vi "期末-7.vi"() -> ()   [LabVIEW 2014]
uses:
  <vilib>/vision/NI_Vision_Development_Module.lvlib
panel:
  in  "紀錄電流":dbl[](array[numeric])
  in  "紀錄中點座標和":bool
  in  "Tab Control 2":enum32{"座標", "座標和", "作圖"}(tab)
  out "瞬間尖點座標":dbl[][](array[numeric])
  out "尖點座標和":dbl[](array[numeric])
  out "填入飽和磁場分量尖點座標和":dbl
  out "相減結果":dbl[](array[numeric])
  out "XY Graph":cluster{"紀錄電流":dbl[], dbl[]}(graph)
  in  "紀錄":bool
  in  "結束實驗":bool
  out "0. 原始畫面":T1(plugin-control)
  in  "1. 範圍選擇":T2={"色相（H）"={0, 255}, "飽和度（S）"={0, 255}, "亮度（L）"={0, 255}} {"亮度（L）" scale=0.0..255.0; "飽和度（S）" scale=0.0..255.0; "色相（H）" scale=0.0..255.0}
  out "Number of Particles":i32
  out "output cluster":cluster{"X":dbl, "Y":dbl}
  in  "Tab Control":T3(tab)
  out "1. 顏色選取":T1(plugin-control)
  out "2. 填補空隙":T1(plugin-control)
  out "4. 形狀修正":T1(plugin-control)
  out "5. 選取結果":T1(plugin-control)
  out "Particle Measurements":dbl[][](array[numeric])
  out "Error Out":errorcluster
  out "滑鼠位置顏色":T4
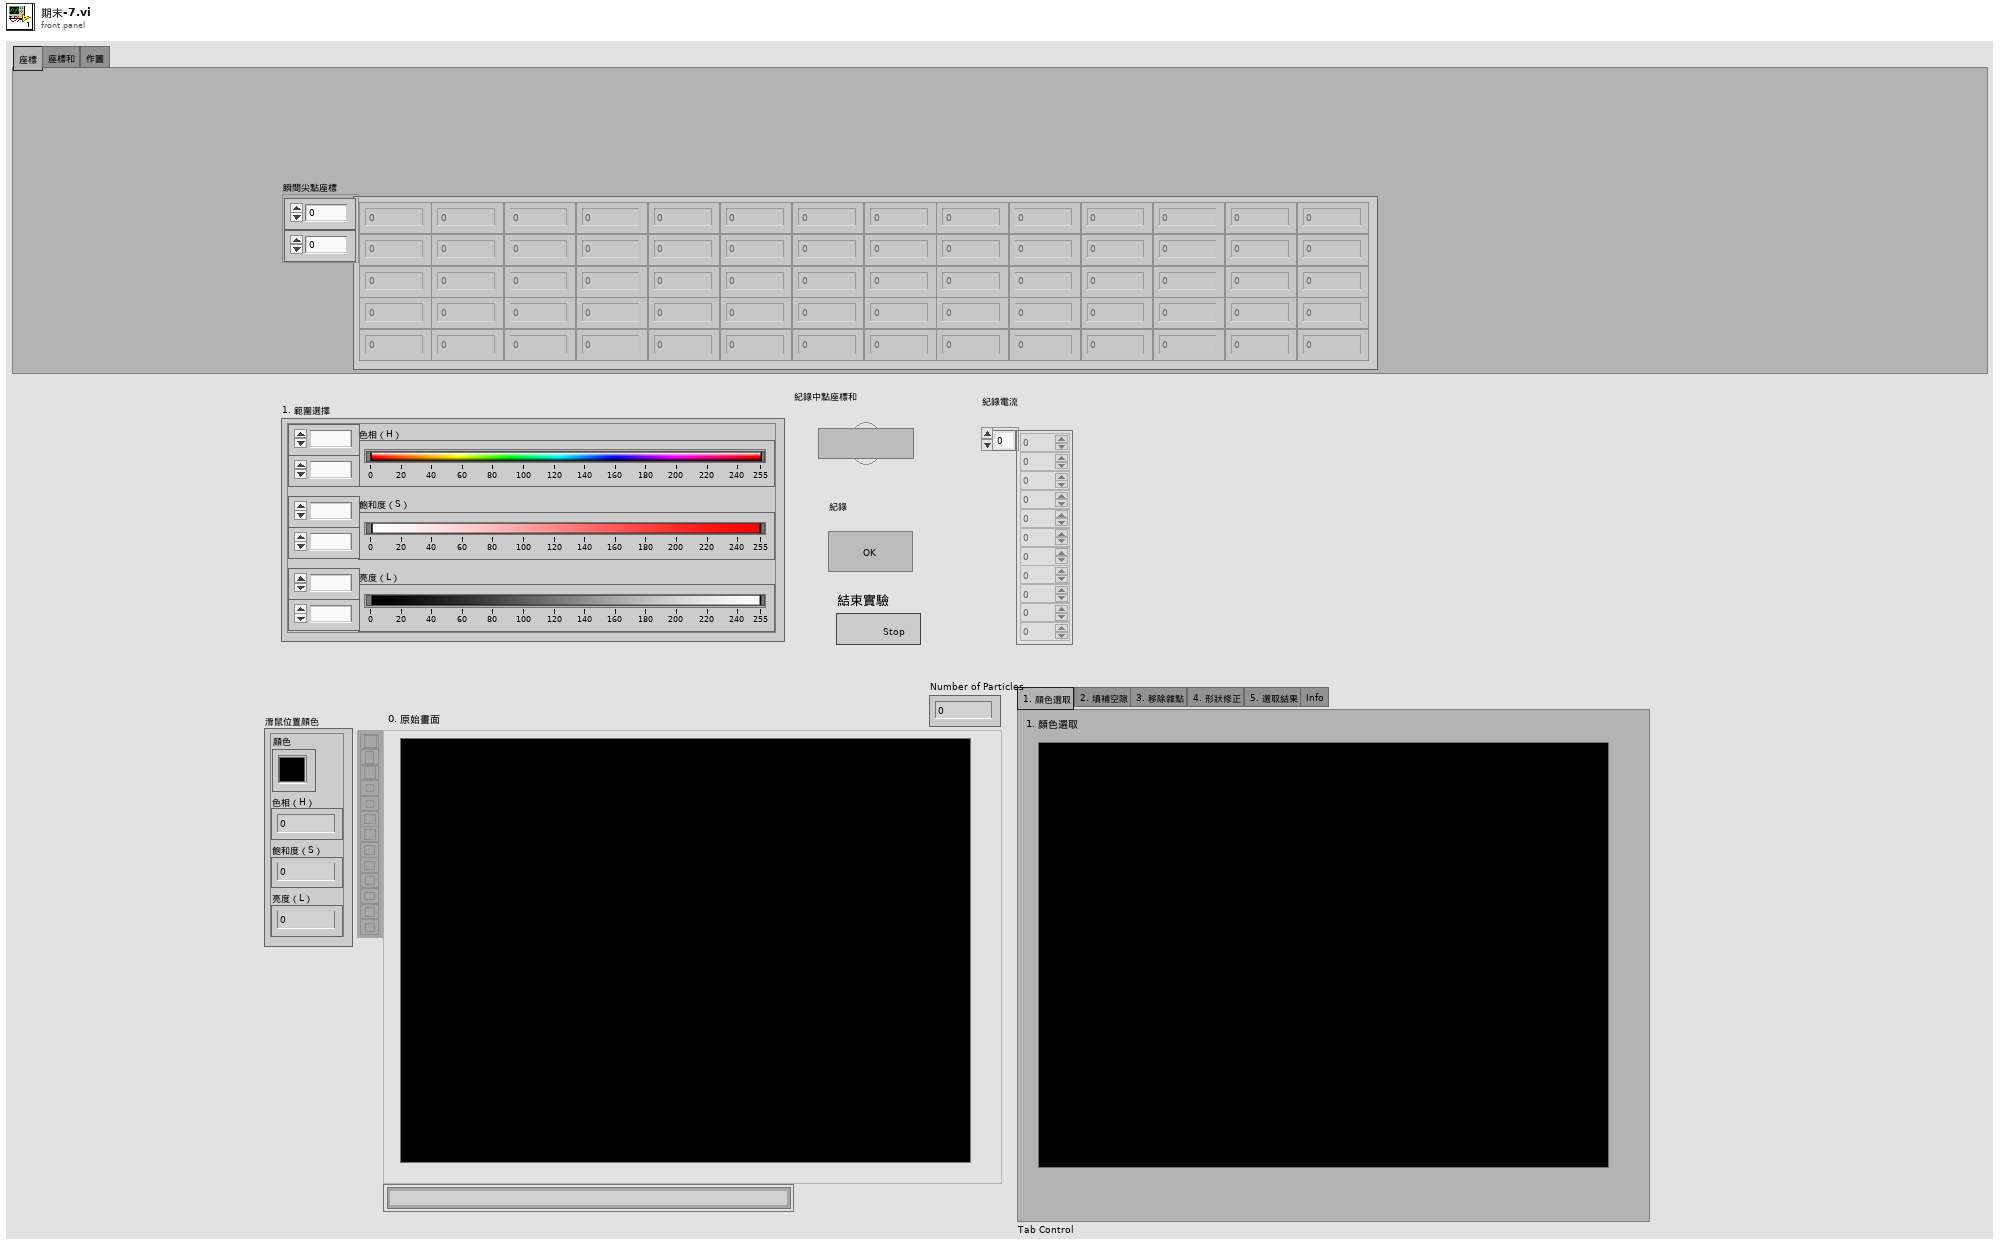
[diagram p1: front panel]
types:
  T1 = typedef "IMAQ Image.ctl" = refnum<image>
  T2 = cluster{"色相（H）":cluster{u8, u8}, "飽和度（S）":cluster{u8, u8}, "亮度（L）":cluster{u8, u8}}
  T3 = enum32{"1. 顏色選取", "2. 填補空隙", "3. 移除雜點", "4. 形狀修正", "5. 選取結果", "Info"}
  T4 = cluster{"色相（H）":u8, "飽和度（S）":u8, "亮度（L）":u8, "顏色":u32}
  T5 = cluster{"Numeric":dbl, "Numeric":dbl, "Numeric":dbl, "Numeric":dbl}
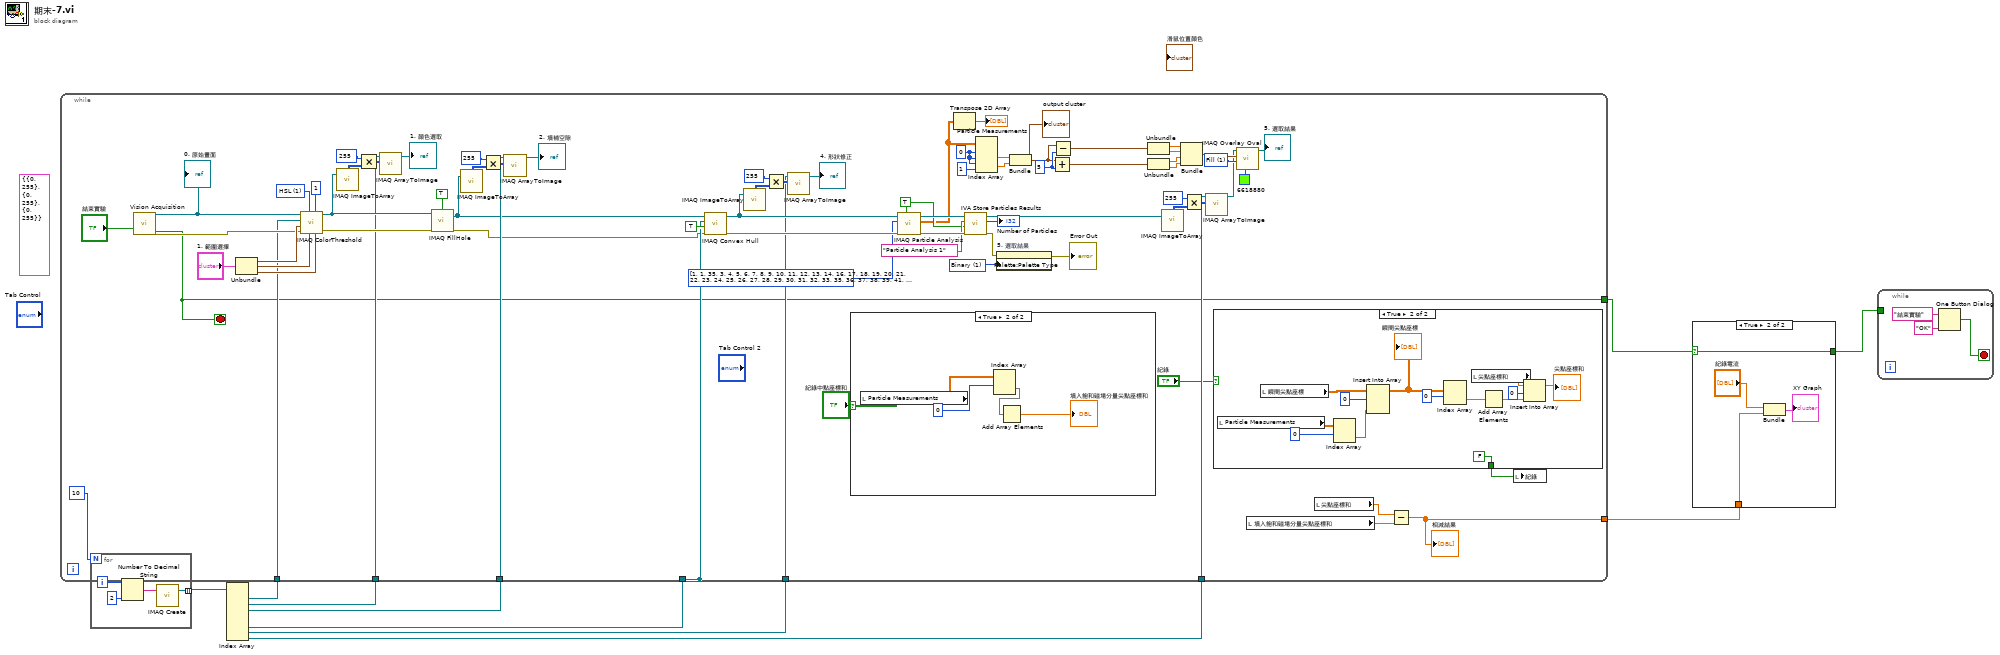
[diagram p0: block diagram]
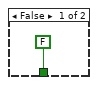
[diagram p4: hidden frame]
diagram:
  (unwired) T2 {"色相（H）"={0, 255}, "飽和度（S）"={0, 255}, "亮度（L）"={0, 255}} ("範圍選擇")
  n1 = for {
    N: 10 -> [_]
    tunnel: [w12] -> w11 mode=indexing
    i -> [w14]
    n2 = Number To Decimal String(number=w14, width (-)=2) -> (decimal integer string=w13:string)
    n3 = call "IMAQ Create"("Image Name"=w13) -> ("New Image"=w12:T1)  [unwired: 4 in, 1 out]
  }
  n4 = Index Array(array=w11) -> (element #1=w10:T1, element #2=w9:T1, element #3=w8:T1, element #6=w6:T1, element #7=w5:T1, element #8=w4:T1)  [unwired: 8 in, 2 out]
  n5 = while {
    tunnel: w8 -> [w58]
    tunnel: w6 -> [w69]
    tunnel: [w69] -> _
    tunnel: w9 -> [w63]
    tunnel: w10 -> [w57]
    tunnel: w5 -> [w51]
    tunnel: w4 -> [w28]
    tunnel: [w22] -> w3
    tunnel: [w16] -> w1
    stop <- w22 stop-if-true
    w33 = u32 1 items=["Frame", "Fill"] ("Drawing Mode (Frame)")
    w42 = 5
    w47 = 0
    w71 = u32 1 items=["Grayscale", "Binary", "Gradient", "Rainbow", "Temperature", "User Defined"] ("Palette")
    w76 = i32[] [1, 1, 35, 3, 4, 5, 6, 7, 8, 9, 10, 11, 12, 13, 14, 16, 17, 18, 19, 20, 21, 22, 23, 24, 25, 26, 27, 28, 29, 30, 31, 32, 33, 35, 36, 37, 38, 39, 41, 42, 43, 45, 46, 48, 49, 50, 51, 53, 54, 55, 56, 58, 59, 60, 61, 62, 63, 64, 65, 66, 68, 69, 70, 71, 72, 73, 74, 75, 76, 77, 78, 79, 80, 81, 82, 83, 84, 85, 86, 87, 88] items=["Center of Mass X", "Center of Mass Y", "First Pixel X", "First Pixel Y", "Bounding Rect Left", "Bounding Rect Top", "Bounding Rect Right", "Bounding Rect Bottom", "Max Feret Diameter Start X", "Max Feret Diameter Start Y", "Max Feret Diameter End X", "Max Feret Diameter End Y", "Max Horiz. Segment Length Left", "Max Horiz. Segment Length Right", "Max Horiz. Segment Length Row", "-", "Bounding Rect Width", "Bounding Rect Height", "Bounding Rect Diagonal", "Perimeter", "Convex Hull Perimeter", "Holes' Perimeter", "Max Feret Diameter", "Equivalent Ellipse Major Axis", "Equivalent Ellipse Minor Axis", "Equivalent Ellipse Minor Axis (Feret)", "Equivalent Rect Long Side", "Equivalent Rect Short Side", "Equivalent Rect Diagonal", "Equivalent Rect Short Side (Feret)", "Average Horiz. Segment Length", "Average Vert. Segment Length", "Hydraulic Radius", "Waddel Disk Diameter", "-", "Area", "Holes' Area", "Particle & Holes' Area", "Convex Hull Area", "Image Area", "-", "Number of Holes", "Number of Horiz. Segments", "Number of Vert. Segments", "-", "Orientation", "Max Feret Diameter Orientation", "-", "% Area/Image Area", "% Area/(Particle & Holes' Area)", "Ratio of Equivalent Ellipse Axes", "Ratio of Equivalent Rect Sides", "-", "Elongation Factor", "Compactness Factor", "Heywood Circularity Factor", "Type Factor", "-", "Sum X", "Sum Y", "Sum XX", "Sum XY", "Sum YY", "Sum XXX", "Sum XXY", "Sum XYY", "Sum YYY", "-", "Moment of Inertia XX", "Moment of Inertia XY", "Moment of Inertia YY", "Moment of Inertia XXX", "Moment of Inertia XXY", "Moment of Inertia XYY", "Moment of Inertia YYY", "Norm. Moment of Inertia XX", "Norm. Moment of Inertia XY", "Norm. Moment of Inertia YY", "Norm. Moment of Inertia XXX", "Norm. Moment of Inertia XXY", "Norm. Moment of Inertia XYY", "Norm. Moment of Inertia YYY", "Hu Moment 1", "Hu Moment 2", "Hu Moment 3", "Hu Moment 4", "Hu Moment 5", "Hu Moment 6", "Hu Moment 7"] ("Pixel Measurements")
    w78 = TRUE ("Connectivity 4/8 (8)")
    w87 = u16 1 items=["RGB", "HSL", "HSV", "HSI"] ("Color Mode")
    n6 = call "Vision Acquisition"("Stop (F)"="結束實驗") -> ("Image Out"=w89:T1, "Stopped"=w22:bool, "error out"=w82:errorcluster)  [unwired: 24 in]
    "0. 原始畫面" <- w89
    n7 = Unbundle("1. 範圍選擇") -> ("色相（H）"=w86:cluster{u8, u8}, "飽和度（S）"=w85:cluster{u8, u8}, "亮度（L）"=w84:cluster{u8, u8})
    n8 = call "IMAQ ColorThreshold"("Blue or Luma or Val or Inten Range"=w84, "Replace Value"=1, "Green or Sat Range"=w85, "Color Mode"=w87, "error in (no error)"=w82, "Red or Hue Range"=w86, "Image Dst"=w57, "Image Src"=w89) -> ("error out"=w73:errorcluster, "Image Dst Out"=w68:T1)  [unwired: 2 out]
    n9 = call "IMAQ ImageToArray"("Image"=w68) -> ("Image Pixels (U8)"=w66:u8[][])  [unwired: 3 in, 4 out]
    n10 = Multiply(x=255, y=w66) -> (x*y=w65:i32[][])
    n11 = call "IMAQ ArrayToImage"("Image Pixels (U8)"=w65, "Image"=w63) -> ("Image Out"=→"1. 顏色選取":T1)  [unwired: 8 in, 1 out]
    n12 = call "IMAQ FillHole"("error in (no error)"=w73, "Image Src"=w68, "Connectivity 4/8 (8)"=TRUE) -> ("error out"=w20:errorcluster, "Image Dst Out"=w21:T1)  [unwired: 1 in, 2 out]
    n13 = call "IMAQ ImageToArray"("Image"=w21) -> ("Image Pixels (U8)"=w61:u8[][])  [unwired: 3 in, 4 out]
    n14 = Multiply(x=255, y=w61) -> (x*y=w62:i32[][])
    n15 = call "IMAQ ArrayToImage"("Image Pixels (U8)"=w62, "Image"=w58) -> ("Image Out"=→"2. 填補空隙":T1)  [unwired: 8 in, 1 out]
    n16 = call "IMAQ Convex Hull"("error in (no error)"=w20, "Connectivity 4/8 (8)"=TRUE, "Image Dst"=w69, "Image Src"=w21) -> ("error out"=w77:errorcluster, "Image Dst Out"=w52:T1)  [unwired: 6 out]
    n17 = call "IMAQ ImageToArray"("Image"=w52) -> ("Image Pixels (U8)"=w55:u8[][])  [unwired: 3 in, 4 out]
    n18 = Multiply(x=255, y=w55) -> (x*y=w56:i32[][])
    n19 = call "IMAQ ArrayToImage"("Image Pixels (U8)"=w56, "Image"=w51) -> ("Image Out"=→"4. 形狀修正":T1)  [unwired: 8 in, 1 out]
    n20 = case shown="True" "紀錄中點座標和" {
      frame False {
      }
      frame True {
        n21 = local read "Particle Measurements"() -> (w92:dbl[][])
        n22 = Index Array(array=w92, index (row)=0) -> (element=w91:dbl[])  [unwired: 1 in]
        n23 = Add Array Elements(numeric array=w91) -> (sum=→"填入飽和磁場分量尖點座標和":dbl)
      }
    }
    n24 = call "IMAQ Particle Analysis"("Connectivity 4/8 (8)"=w78, "error in (no error)"=w77, "Pixel Measurements"=w76, "Image"=w52) -> ("error out"=w81:errorcluster, "Particle Measurements (Pixels)"=w48:dbl[][], "Image Out (duplicate)"=w79:T1)  [unwired: 1 in, 4 out]
    n25 = Transpose 2D Array(2D array=w48) -> (transposed array=→"Particle Measurements":dbl[][])
    n26 = call <vilib>:"IVA Store Particles Results.vi"("error in (no error)"=w81, "Connectivity 4/8 (8)"=w78, "Step Name"="Particle Analysis 1", "Image in"=w79) -> ("error out"=w72:errorcluster, "Number of Particles"=→"Number of Particles":i32, "Image dup"=w32:T1)  [unwired: 5 out]
    n27 = Index Array(array=w48, index (row) #1=w47, index (col) #1=w47, index (row) #2=w47, index (col) #2=1) -> (element #1=w45:dbl, element #2=w44:dbl)
    n28 = property on="5. 選取結果" class="ImageControl"(error in=w72, "Palette:Palette Type"=w71) -> (error out=→"Error Out":errorcluster)  [unwired: 1 in, 1 out]
    n29 = Bundle("Numeric"=w45, "Numeric"=w44) -> (w41:cluster{"Numeric":dbl, "Numeric":dbl})  [unwired: 1 in]
    "output cluster" <- w41
    n30 = Add(x=w41, y=w42) -> (x+y=w39:cluster{"Numeric":dbl, "Numeric":dbl})
    n31 = Subtract(x=w41, y=w42) -> (x-y=w40:cluster{"Numeric":dbl, "Numeric":dbl})
    n32 = Unbundle(w40) -> ("Numeric"=w38:dbl, "Numeric"=w37:dbl)
    n33 = Unbundle(w39) -> ("Numeric"=w36:dbl, "Numeric"=w35:dbl)
    n34 = call "IMAQ ImageToArray"("Image"=w32) -> ("Image Pixels (U8)"=w29:u8[][])  [unwired: 3 in, 4 out]
    n35 = Bundle("Numeric"=w38, "Numeric"=w37, "Numeric"=w36, "Numeric"=w35) -> (w34:T5)  [unwired: 1 in]
    n36 = Multiply(x=255, y=w29) -> (x*y=w30:i32[][])
    n37 = call "IMAQ ArrayToImage"("Image Pixels (U8)"=w30, "Image"=w28) -> ("Image Out"=w27:T1)  [unwired: 8 in, 1 out]
    n38 = case shown="True" "紀錄" {
      tunnel: [FALSE FALSE] -> w23
      frame False {
      }
      frame True {
        n39 = local read "Particle Measurements"() -> (w97:dbl[][])
        n40 = local read "瞬間尖點座標"() -> (w103:dbl[][])
        n41 = Index Array(array=w97, index (row)=0) -> (element=w102:dbl[])  [unwired: 1 in]
        n42 = Insert Into Array(array=w103, index (row)=0 ("index"), new element=w102) -> (w105:dbl[][])  [unwired: 1 in]
        "瞬間尖點座標" <- w105
        n43 = Index Array(array=w105, index (row)=0) -> (element=w107:dbl[])  [unwired: 1 in]
        n44 = local read "尖點座標和"() -> (w98:dbl[])
        n45 = Add Array Elements(numeric array=w107) -> (sum=w100:dbl)
        n46 = Insert Into Array(array=w98, index=0 ("index (row)"), new element=w100) -> (→"尖點座標和":dbl[])
      }
    }
    n47 = call "IMAQ Overlay Oval"("Color"=u32 6618880, "Drawing Mode (Frame)"=w33, "Bounding Rectangle"=w34, "Image"=w27) -> ("Image Out"=→"5. 選取結果":T1)  [unwired: 6 in, 1 out]
    n48 = local read "填入飽和磁場分量尖點座標和"() -> (w17:dbl)
    n49 = local read "尖點座標和"() -> (w18:dbl[])
    n50 = Subtract(x=w18, y=w17) -> (x-y=w16:dbl[])
    "相減結果" <- w16
    n51 = local write "紀錄"(w23) -> ()
  }
  n52 = case shown="True" w3 {
    selector: w3 -> [w108 w112]
    tunnel: [w108 w112] -> w2
    tunnel: w1 -> [_ w111]
    frame False {
    }
    frame True {
      n53 = Bundle("紀錄電流"="紀錄電流", w111) -> (→"XY Graph":cluster{"紀錄電流":dbl[], dbl[]})  [unwired: 1 in]
    }
  }
  n54 = while {
    tunnel: w2 -> [_]
    stop <- w115 stop-if-true
    n55 = One Button Dialog(message="結束實驗", button name ("OK")="OK") -> (true=w115:bool)
  }
